vi "SentinelController v33.vi"() -> ()   [LabVIEW 2011] (continued)
                                n3481 = local write "H2 binning string hid"(w2946) -> ()
                                }
                                frame #2 {
                                n3482 = local read "VISA bus 2 resource name out hid"() -> (w2955:refnum<visa-resource-name>)
                                n3483 = local read "VISA bus 2 error out hid"() -> (w2956:errorcluster)
                                n3484 = local read "H2 binning string hid"() -> (w2949:string)
                                n3485 = local read "GPIB bus 2 traffic"() -> (w2953:string)
                                n3486 = VISA Write(VISA resource name=w2955, write buffer=w2949, error in (no error)=w2956) -> (VISA resource name out=w2948:refnum<visa-resource-name>, error out=w2947:errorcluster)  [unwired: 1 out]
                                n3487 = local write "VISA bus 2 error out hid"(w2947) -> ()
                                n3488 = Unbundle By Name(w2947) -> ("status"=w2954:bool)
                                n3489 = Concatenate Strings(w2953, "\r\n", "Bus 2 write: " ("string"), w2949) -> (w2951:string)
                                n3490 = local write "GPIB bus 2 traffic"(w2951) -> ()
                                n3491 = local write "GPIB bus 2 write error"(w2954) -> ()
                                }
                                frame #3 {
                                n3492 = while {
                                tunnel: w2959 -> [w2965]
                                tunnel: w2958 -> [w2964]
                                tunnel: [w2960] -> w2957
                                stop <- w2961 stop-if-true
                                n3493 = local read "GPIB bus 2 traffic"() -> (w2967:string)
                                n3494 = VISA Read(VISA resource name=w2965, byte count=u32 256, error in (no error)=w2964) -> (VISA resource name out=w2972:refnum<visa-resource-name>, read buffer=w2960:string, error out=w2971:errorcluster)  [unwired: 1 out]
                                n3495 = local write "VISA bus 2 resource name out hid"(w2972) -> ()
                                n3496 = Unbundle By Name(w2971) -> ("status"=w2966:bool)
                                n3497 = Match True/False String(2:"false string" ("false string"), 3:"ECHO:", 4:w2960) -> (0:w2961:bool)  [unwired: 1 out]
                                n3498 = local write "GPIB bus 2 read error"(w2966) -> ()
                                n3499 = Concatenate Strings(w2967, "\r\n", "Bus 2 read: " ("string"), w2960) -> (w2969:string)
                                n3500 = local write "GPIB bus 2 traffic"(w2969) -> ()
                                }
                                }
                                frame #4 {
                                n3501 = local read "GPIB bus 2 read error"() -> (w2974:bool)
                                n3502 = case shown="False" w2974 {
                                tunnel: w2975 -> [w2976 _]
                                frame False {
                                n3503 = local write "H2 echo hid"(w2976) -> ()
                                n3504 = local read "H2 binning string hid"() -> (w2977:string)
                                n3505 = Equal?(x=w2977, y=w2976) -> (x = y?=w2978:bool)
                                n3506 = case shown="True" w2978 {
                                frame False {
                                n3507 = local write "NS6040 tester states H2 hid"(SC_NS6040_tester_states."sending ECHONG" ("NS6040 tester states H2 hid")) -> ()
                                }
                                frame True {
                                n3508 = local write "NS6040 tester states H2 hid"(SC_NS6040_tester_states."sending ECHOOK" ("NS6040 tester states H2 hid")) -> ()
                                }
                                }
                                }
                                frame True {
                                n3509 = flat-sequence {
                                frame #0 {
                                n3510 = while {
                                stop <- w2982 stop-if-true
                                n3511 = Wait (ms)(milliseconds to wait=u32 100) -> ()  [unwired: 1 out]
                                n3512 = One Button Dialog(message="Echo readback error for H2.\nClosing Bus 2.", button name ("OK")="Dismiss") -> (true=w2982:bool)
                                }
                                }
                                frame #1 {
                                n3513 = local write "NS6040 tester states H2 hid"(SC_NS6040_tester_states."closing bus" ("NS6040 tester states H1 hid")) -> ()
                                }
                                }
                                }
                                }
                                }
                                }
                                }
                                frame "sending ECHONG" {
                                n3514 = flat-sequence {
                                frame #0 {
                                w2986 = "ECHONG\n"
                                n3515 = local read "VISA bus 2 resource name out hid"() -> (w2993:refnum<visa-resource-name>)
                                n3516 = local read "VISA bus 2 error out hid"() -> (w2994:errorcluster)
                                n3517 = local read "GPIB bus 2 traffic"() -> (w2991:string)
                                n3518 = VISA Write(VISA resource name=w2993, write buffer=w2986, error in (no error)=w2994) -> (error out=w2987:errorcluster)  [unwired: 2 out]
                                n3519 = local write "VISA bus 2 error out hid"(w2987) -> ()
                                n3520 = Unbundle By Name(w2987) -> ("status"=w2992:bool)
                                n3521 = Concatenate Strings(w2991, "\r\n", "Bus 2 write: " ("string"), w2986) -> (w2989:string)
                                n3522 = local write "GPIB bus 2 traffic"(w2989) -> ()
                                n3523 = local write "GPIB bus 2 write error"(w2992) -> ()
                                }
                                frame #1 {
                                n3524 = while {
                                stop <- w2995 stop-if-true
                                n3525 = Wait (ms)(milliseconds to wait=u32 100) -> ()  [unwired: 1 out]
                                n3526 = One Button Dialog(message="ECHO from handler 2 did not match BINON'\nError message from \"sending ECHONG\" state\nBINON message will be resent.") -> (true=w2995:bool)  [unwired: 1 in]
                                }
                                }
                                frame #2 {
                                n3527 = local write "NS6040 tester states H2 hid"(SC_NS6040_tester_states."sending BINON?" ("NS6040 tester states H1 hid")) -> ()
                                }
                                }
                                }
                                frame "sending ECHOOK" {
                                n3528 = flat-sequence {
                                frame #0 {
                                w2999 = "ECHOOK\n"
                                n3529 = local read "VISA bus 2 resource name out hid"() -> (w3006:refnum<visa-resource-name>)
                                n3530 = local read "VISA bus 2 error out hid"() -> (w3007:errorcluster)
                                n3531 = local read "GPIB bus 2 traffic"() -> (w3004:string)
                                n3532 = VISA Write(VISA resource name=w3006, write buffer=w2999, error in (no error)=w3007) -> (error out=w3000:errorcluster)  [unwired: 2 out]
                                n3533 = local write "VISA bus 2 error out hid"(w3000) -> ()
                                n3534 = Unbundle By Name(w3000) -> ("status"=w3005:bool)
                                n3535 = Concatenate Strings(w3004, "\r\n", "Bus 2 write: " ("string"), w2999) -> (w3002:string)
                                n3536 = local write "GPIB bus 2 traffic"(w3002) -> ()
                                n3537 = local write "GPIB bus 2 write error"(w3005) -> ()
                                }
                                frame #1 {
                                n3538 = Tick Count (ms)() -> (millisecond timer value=w3009:u32)
                                n3539 = Tick Count (ms)() -> (millisecond timer value=w3010:u32)
                                n3540 = local write "H2 Ready with sites"(FALSE ("waiting")) -> ()
                                n3541 = local write "H2 Testing"(FALSE ("waiting")) -> ()
                                n3542 = local write "H2 Indexing"(TRUE ("waiting")) -> ()
                                n3543 = local write "H2 tt end hidden"(w3009) -> ()
                                n3544 = local write "H2 it start hidden"(w3010) -> ()
                                }
                                frame #2 {
                                n3545 = local read "H2 tt start hidden"() -> (w3016:u32)
                                n3546 = local read "H2 tt end hidden"() -> (w3017:u32)
                                n3547 = Subtract(x=w3017, y=w3016) -> (x-y=w3015:u32)
                                n3548 = Divide(x=w3015, y=u32 1000) -> (x/y=w3013:dbl)
                                n3549 = local write "H2 measured Test Time"(w3013) -> ()
                                }
                                frame #3 {
                                n3550 = local read "H2 binning string hid"() -> (w3018:string)
                                n3551 = local read "H2 FULLSITES? binary hid"() -> (w3035:string)
                                n3552 = String Subset(string=w3018, offset (0)=6, length (rest)=35 ("length (rest)")) -> (substring=w3032:string)
                                n3553 = local read "H2 Device Count"() -> (w3020:u32)
                                n3554 = local read "H2 Good Units"() -> (w3022:u32)
                                n3555 = Search and Replace String(replace all?=TRUE ("replace all? (F)"), input string=w3032, search string=",") -> (result string=w3026:string)  [unwired: 5 in, 3 out]
                                n3556 = Search and Replace String(replace all?=TRUE ("replace all? (F)"), input string=w3035, search string="1") -> (number of replacements=w3036:i32)  [unwired: 5 in, 3 out]
                                n3557 = Add(x=w3036, y=w3020) -> (x+y=w3019:u32)
                                n3558 = Divide(x=w3022, y=w3020) -> (x/y=w3025:dbl)
                                n3559 = Search and Replace String(replace all?=TRUE ("replace all? (F)"), input string=w3026, search string="1") -> (number of replacements=w3027:i32)  [unwired: 5 in, 3 out]
                                n3560 = local write "H2 Device Count"(w3019) -> ()
                                n3561 = Add(x=w3027, y=w3022) -> (x+y=w3021:u32)
                                n3562 = Multiply(x=w3025, y=100.0) -> (x*y=w3023:dbl)
                                n3563 = local write "H2 Good Units"(w3021) -> ()
                                n3564 = local write "H2 cycle yield hid"(w3023) -> ()
                                }
                                frame #4 {
                                n3565 = local read "H2 Device Count"() -> (w3039:u32)
                                n3566 = local read "H2 Good Units"() -> (w3040:u32)
                                n3567 = Divide(x=w3040, y=w3039) -> (x/y=w3043:dbl)
                                n3568 = Multiply(x=w3043, y=100.0) -> (x*y=w3041:dbl)
                                n3569 = local write "H2 lot yield mon"(w3041) -> ()
                                }
                                frame #5 {
                                n3570 = local write "NS6040 tester states H2 hid"(SC_NS6040_tester_states."serial polling handler" ("NS6040 tester states H2 hid")) -> ()
                                }
                                }
                                }
                                frame "closing bus" {
                                n3571 = local read "GPIB bus 2 traffic"() -> (w3049:string)
                                n3572 = local write "Exit SC tester H2 StMach hid"(TRUE ("Exit H2 state machine hid")) -> ()
                                n3573 = local read "VISA bus 2 resource name out hid"() -> (w3053:refnum<visa-resource-name>)
                                n3574 = local read "VISA bus 2 error out hid"() -> (w3052:errorcluster)
                                n3575 = Concatenate Strings(w3049, "\r\n", "Bus 2: closing " ("string")) -> (w3047:string)
                                n3576 = local write "GPIB bus 2 traffic"(w3047) -> ()
                                n3577 = VISA Close(VISA resource name=w3053, error in (no error)=w3052) -> (error out=w3051:errorcluster)
                                n3578 = Unbundle By Name(w3051) -> ("status"=w3050:bool)
                                n3579 = local write "VISA bus 2 close error"(w3050) -> ()
                                }
                                }
                              }
                              frame #1 {
                                n3580 = local read "Slow for  Diagnostics"() -> (w3054:bool)
                                n3581 = case shown="True" w3054 {
                                frame False {
                                }
                                frame True {
                                n3582 = local read "GPIB wait time (ms)"() -> (w3055:u32)
                                n3583 = Wait (ms)(milliseconds to wait=w3055) -> ()  [unwired: 1 out]
                                }
                                }
                              }
                            }
                            n3584 = local read "Exit SC tester H2 StMach hid"() -> (w2742:bool)
                          }
                        }
                      }
                    }
                  }
                }
              }
              n3585 = local read "POWER"() -> (w2197:bool)
            }
          }
        }
      }
    }
  }
